vi "IOCtest.vi"() -> ()   [LabVIEW 2018]
uses:
  <userlib>/caLab/PV.ctl
  <userlib>/caLab/Private/Put_I32_PV.vi
panel:
  out "Waveform Chart":dbl(graph)
  in  "stop":bool
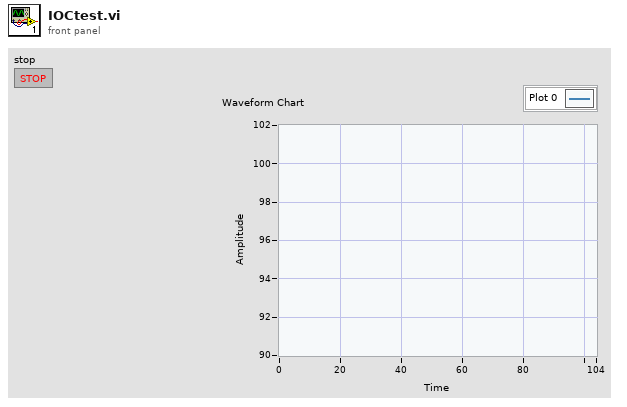
[diagram p1: front panel]
types:
  T1 = typedef "PV.ctl" = cluster{"PV Name":string, "Data Type":string, "Fields":cluster{"Field Name":string, "Field Value":string}[]}[]
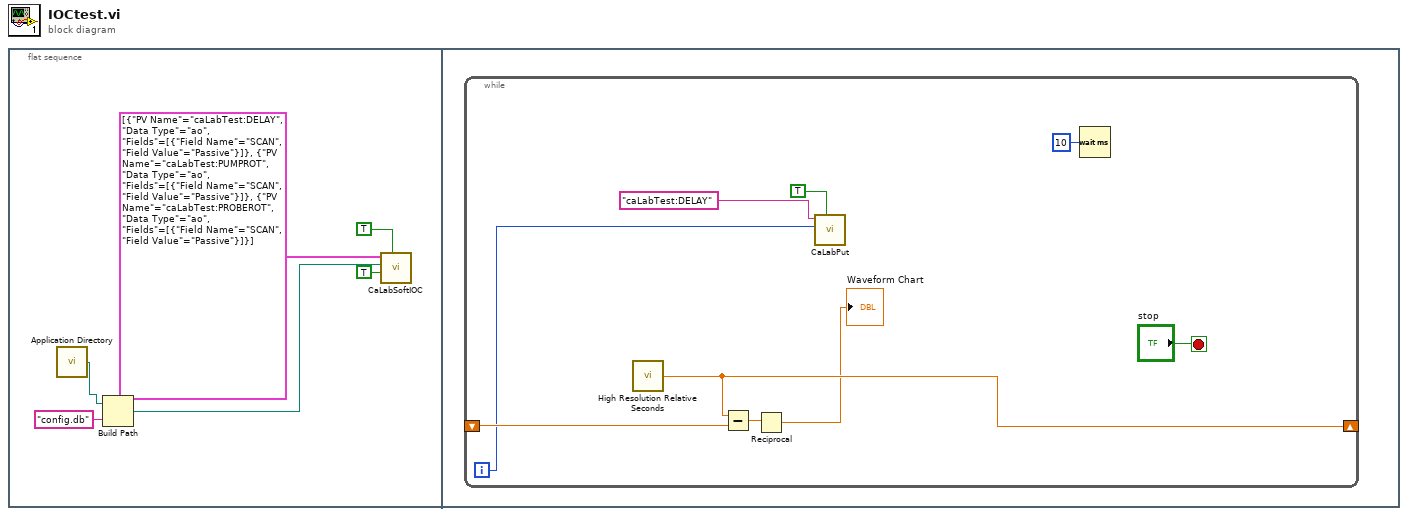
[diagram p0: block diagram]
diagram:
  n1 = flat-sequence {
    frame #0 {
      n2 = call <vilib>:"Application Directory.vi"() -> ("Application Directory"=w1:path)
      n3 = Build Path(base path=w1, name or relative path="config.db") -> (appended path=w2:path)
      n4 = call <userlib>:"CaLabSoftIOC.vi"("Minimize IOC"=TRUE, "Force"=TRUE, "Config File"=w2, "PV set"=T1 [{"PV Name"="caLabTest:DELAY", "Data Type"="ao", "Fields"=[{"Field Name"="SCAN", "Field Value"="Passive"}]}, {"PV Name"="caLabTest:PUMPROT", "Data Type"="ao", "Fields"=[{"Field Name"="SCAN", "Field Value"="Passive"}]}, {"PV Name"="caLabTest:PROBEROT", "Data Type"="ao", "Fields"=[{"Field Name"="SCAN", "Field Value"="Passive"}]}]) -> ()  [unwired: 2 in, 4 out]
    }
    frame #1 {
      n5 = while {
        shift-right: [w13] -> _
        shift-left: _ -> [w12]
        i -> [w9]
        stop <- "stop" stop-if-true
        n6 = call <vilib>:"High Resolution Relative Seconds.vi"() -> ("relative seconds"=w13:dbl)
        n7 = Subtract(x=w13, y=w12) -> (x-y=w11:dbl)
        n8 = Reciprocal(x=w11) -> (1/x=→"Waveform Chart":dbl)
        n9 = call-poly <userlib>:"CaLabPut.vi"("Synchronous (F)"=TRUE, "Value"=w9, "PV Name"="caLabTest:DELAY") -> ()  [unwired: 5 in, 4 out]
        n10 = Wait (ms)(milliseconds to wait=u32 10) -> ()  [unwired: 1 out]
      }
    }
  }
